vi "OE2052_Data Index.vi"(1 "Parameter Type":u16(ring) items=["Demod 1_X", "Demod 1_Y", "Demod 1_R", "Demod 1_θ", "Demod 1_Frequency", "Demod 2_X", "Demod 2_Y", "Demod 2_R", "Demod 2_θ", "Demod 2_Frequency", "Demod 3_X", "Demod 3_Y", "Demod 3_R", "Demod 3_θ", "Demod 3_Frequency", "Demod 4_X", "Demod 4_Y", "Demod 4_R", "Demod 4_θ", "Demod 4_Frequency", "Demod 1_X_Noise", "Demod 2_X_Noise", "SIGIN 1_ADC", "SIGIN 2_ADC", "SIGIN 1_LF ADC", "SIGIN 2_LF ADC"], 2 "Input Date Array":dbl[](array[numeric])) -> (0 "Parameter":dbl)   [LabVIEW 2011]
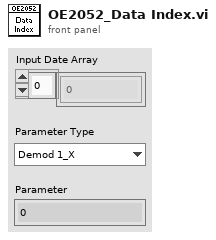
[diagram p1: front panel]
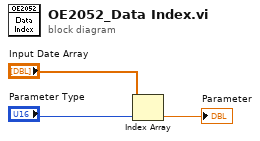
[diagram p0: block diagram]
diagram:
  n1 = Index Array(array="Input Date Array", index="Parameter Type") -> (element=→"Parameter":dbl)
